vi "数据库查询.vi"(5 "condition":string, 7 "columns":string[](array[string]), 8 "error in (no error)":errorcluster, 11 "table":string) -> (0 "error out":errorcluster, 2 "columns 2":string[](array[string]), 3 "data":variant[][](array[variant]))   [LabVIEW 2016, in "Alarm interface.lvlib"]
uses:
  Alarm interface.lvlib
  <vilib>/addons/database/Connection.llb/DB Tools Open Connec (String).vi
  <vilib>/addons/database/NI_Database_API.lvlib
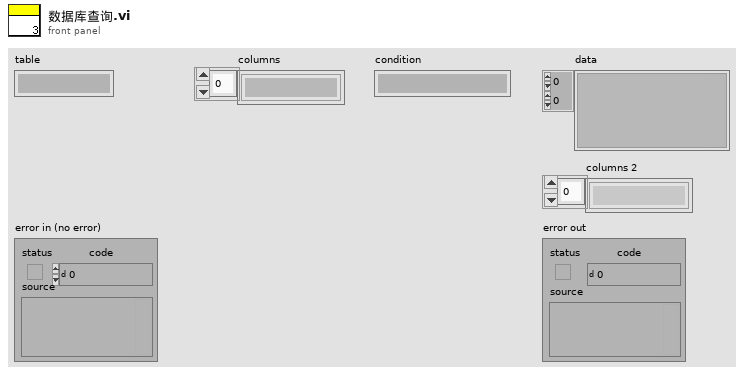
[diagram p1: front panel]
types:
  T1 = typedef "NI_Database_API.lvlib/Conn ObjectReference.ctl" = refnum<k1>
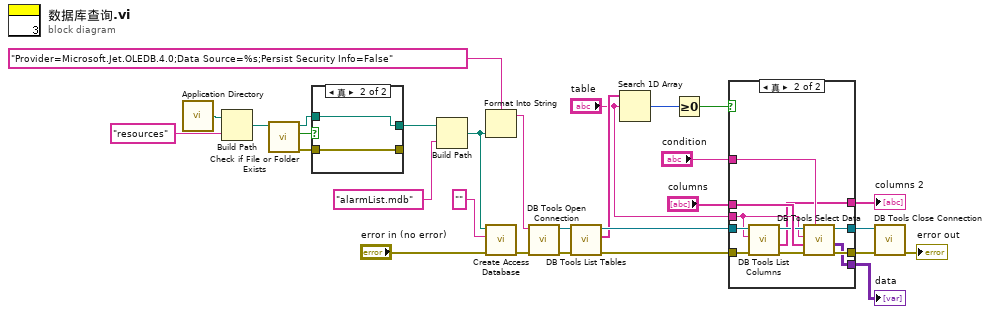
[diagram p0: block diagram]
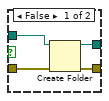
[diagram p3: hidden frame]
diagram:
  n1 = call <vilib>:"Application Directory.vi"() -> ("Application Directory"=w25:path)
  n2 = Build Path(base path=w25, name or relative path="resources" ("名称或相对路径")) -> (appended path=w23:path)
  n3 = call <vilib>:"Check if File or Folder Exists.vi"("path"=w23) -> ("error out"=w20:errorcluster, "file or folder exists?"=w22:bool, "dup path"=w21:path)  [unwired: 8 in]
  n4 = case shown="真" w22 {
    tunnel: [w30 w35] -> w19
    tunnel: w21 -> [w33 w35]
    tunnel: w20 -> [w32 w34]
    tunnel: [w31 w34] -> _
    frame False {
      n5 = Create Folder(path (use dialog)=w33, error in=w32) -> (created path=w30:path, error out=w31:errorcluster)  [unwired: 1 in, 1 out]
    }
    frame True {
    }
  }
  n6 = Build Path(base path=w19, name or relative path="alarmList.mdb" ("名称或相对路径")) -> (appended path=w17:path)
  n7 = Format Into String(format string="Provider=Microsoft.Jet.OLEDB.4.0;Data Source=%s;Persist Security Info=False", w17) -> (resulting string=w28:string)  [unwired: 2 in, 1 out]
  n8 = call "Create Access Database.vi"("错误输入（无错误）"="error in (no error)", "Password"="", "路径"=w17) -> ("错误输出"=w27:errorcluster)  [unwired: 8 in]
  n9 = call-poly <vilib>:"DB Tools Open Connection.vi"("error in (no error)"=w27, "connection information"=w28) -> ("error out"=w14:errorcluster, "connection reference"=w7:T1)  [unwired: 6 in]
  n10 = call <vilib>:"DB Tools List Tables.vi"("error in (no error)"=w14, "connection reference"=w7) -> ("error out"=w8:errorcluster, "tables"=w5:string[], "connection reference out"=w6:T1)  [unwired: 3 in]
  n11 = Search 1D Array(1D array=w5, element="table") -> (index of element=w3:i32)  [unwired: 1 in]
  n12 = Greater Or Equal To 0?(x=w3) -> (x >= 0?=w2:bool)
  n13 = case shown="真" w2 {
    tunnel: [w37 w48] -> w13
    tunnel: [w36 w47] -> w12
    tunnel: "condition" -> [_ w46]
    tunnel: "columns" -> [_ w45]
    tunnel: [_ w44] -> w9
    tunnel: w8 -> [w36 w41]
    tunnel: w6 -> [w37 w40]
    tunnel: "table" -> [_ w39]
    tunnel: [_ w38] -> w1
    frame False {
    }
    frame True {
      n14 = call <vilib>:"DB Tools List Columns.vi"("error in (no error)"=w41, "table"=w39, "connection reference"=w40) -> ("error out"=w43:errorcluster, "columns"=w38:string[], "connection reference out"=w42:T1)  [unwired: 1 in, 1 out]
      n15 = call <vilib>:"DB Tools Select Data.vi"("condition"=w46, "error in (no error)"=w43, "columns"=w45, "table"=w39, "connection reference"=w42) -> ("error out"=w47:errorcluster, "data"=w44:variant[][], "connection reference out"=w48:T1)  [unwired: 1 in]
    }
  }
  "data" <- w9
  "columns 2" <- w1
  n16 = call <vilib>:"DB Tools Close Connection.vi"("error in (no error)"=w12, "connection reference"=w13) -> ("error out"=→"error out":errorcluster)  [unwired: 5 in]
